vi "AutonomousScript_CommandAndControl.vi"() -> ()   [LabVIEW 2015]
panel:
  out "current command":string
  out "Script":string="drive .3 .4 .0\nwait 2000\nstop\nwait 3000\ndrive .1 .2 .3\nwait 5000\nstop\nwait 1000\nlift .75\nwait 3600\nstop\n\n"
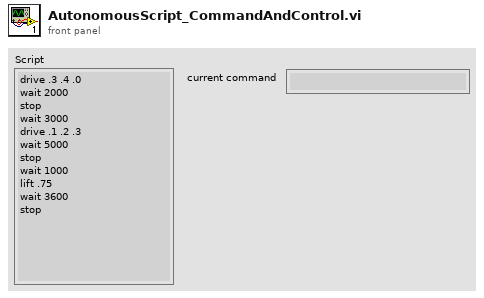
[diagram p1: front panel]
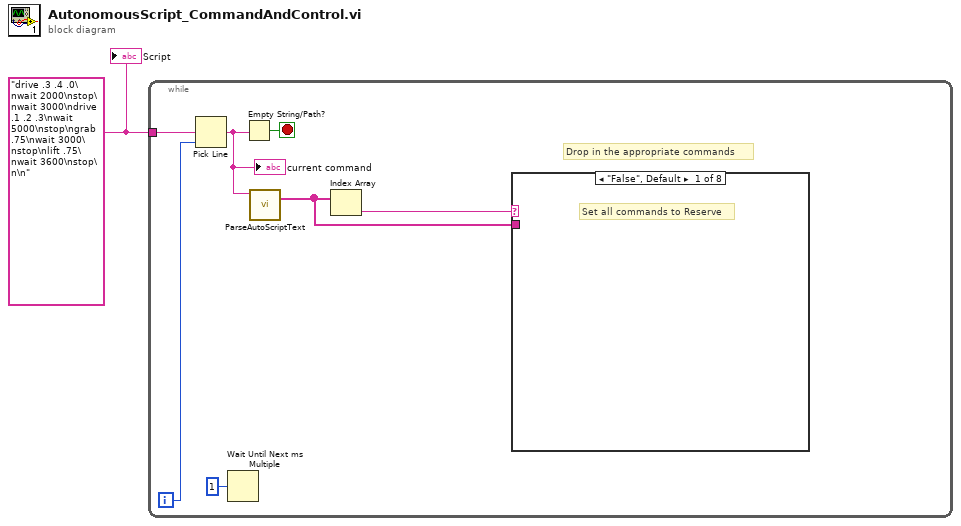
[diagram p0: block diagram]
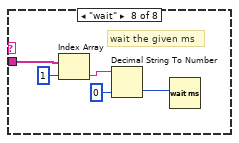
[diagram p8: hidden frame]
diagram:
  w1 = "drive .3 .4 .0\nwait 2000\nstop\nwait 3000\ndrive .1 .2 .3\nwait 5000\nstop\ngrab .75\nwait 3000\nstop\nlift .75\nwait 3600\nstop\n\n"
  n1 = while {
    tunnel: w1 -> [w7]
    i -> [w8]
    stop <- w6 stop-if-true
    # "Drop in the appropriate commands"
    n2 = Pick Line(multi-line string=w7, line index=w8) -> (output string=w5:string)  [unwired: 1 in]
    "current command" <- w5
    n3 = Wait Until Next ms Multiple(millisecond multiple=u32 1) -> ()  [unwired: 1 out]
    n4 = Empty String/Path?(string/path=w5) -> (empty?=w6:bool)
    n5 = call "ParseAutoScriptText.vi"("output string"=w5) -> ("Array"=w2:string[])  [unwired: 10 in]
    n6 = Index Array(array=w2) -> (element=w3:string)  [unwired: 1 in]
    n7 = case shown="\"False\", Default" w3 {
      tunnel: w2 -> [_ _ _ _ _ _ _ w10]
      frame "False", Default {
        # "Set all commands to Reserve"
      }
      frame "drive" {
        # "distance\nspeed"
      }
      frame "dfd" {
        # "distance\nspeed"
      }
      frame "dft" {
      }
      frame "turn" {
        # "Turn x degrees"
      }
      frame "shoot" {
        # "start the shoot sequence"
      }
      frame "wedge" {
        # "Command the wedge up or down"
      }
      frame "wait" {
        # "wait the given ms"
        n8 = Index Array(array=w10, index=1) -> (element=w12:string)
        n9 = Decimal String To Number(string=w12, default (0L)=u32 0 ("default (0 I32)")) -> (number=w9:u32)  [unwired: 1 in, 1 out]
        n10 = Wait (ms)(milliseconds to wait=w9) -> ()  [unwired: 1 out]
      }
    }
  }
  "Script" <- w1
